vi "find_fiducial_test.vi"() -> ()   [LabVIEW 2019]
uses:
  gVision/gVision.lvlib
  <vilib>/vision/NI_Vision_Development_Module.lvlib
panel:
  out "error out":errorcluster
  out "coords":cluster{"x":dbl, "y":dbl}[](array[cluster])
  out "Image":T1(plugin-control)
  in  "interactive":bool
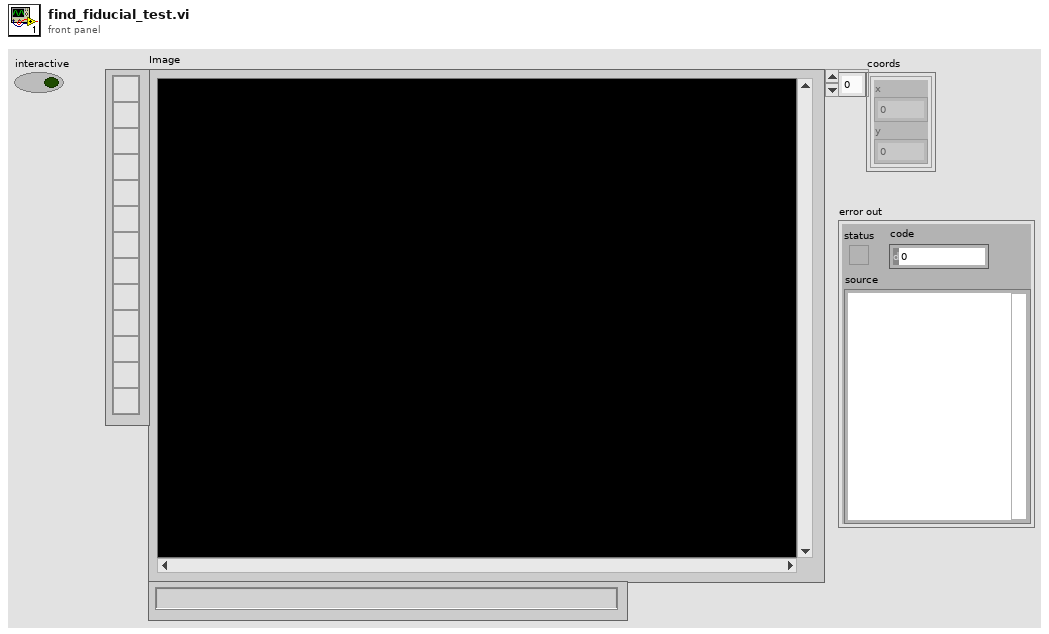
[diagram p1: front panel]
types:
  T1 = typedef "IMAQ Image.ctl" = refnum<image>
  T2 = typedef "Image Type" = u32
  T3 = cluster{"shrinkFactor":sgl, "dilateSize":i32, "sizeMin":sgl, "sizeMax":sgl, "arMin":sgl, "arMax":sgl, "colorGroups":i32, "maxAttempts":i32}
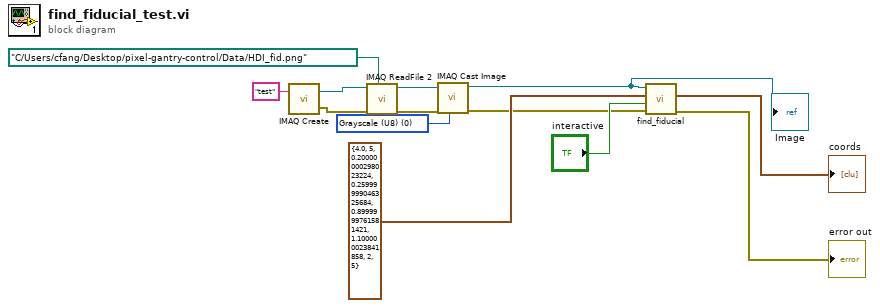
[diagram p0: block diagram]
diagram:
  w1 = T2 0 items=["Grayscale (U8)", "Grayscale (I16)", "Grayscale (SGL)", "Complex (CSG)", "RGB (U32)", "HSL (U32)", "RGB (U64)", "Grayscale (U16)"] ("Image Type")
  n1 = call "IMAQ Create"("Image Name"="test") -> ("New Image"=w11:T1, "error out"=w9:errorcluster)  [unwired: 4 in]
  n2 = call "IMAQ ReadFile 2"("File Path"=path "C:/Users/cfang/Desktop/pixel-gantry-control/Data/HDI_fid.png", "error in (no error)"=w9, "Image"=w11) -> ("error out"=w5:errorcluster, "Image Out"=w3:T1)  [unwired: 4 in, 3 out]
  n3 = call "IMAQ Cast Image"("Image Type"=w1, "error in (no error)"=w5, "Image Src"=w3) -> ("error out"=w4:errorcluster, "Image Dst Out"=w2:T1)  [unwired: 7 in]
  "Image" <- w2
  n4 = call "find_fiducial.vi"("error in"=w4, "interactive"="interactive", "Fiducial Parameters"=T3 {"shrinkFactor"=4.0, "dilateSize"=5, "sizeMin"=0.2, "sizeMax"=0.26, "arMin"=0.9, "arMax"=1.1, "colorGroups"=2, "maxAttempts"=5}, "Image"=w2) -> ("error out"=→"error out":errorcluster, "coords"=→"coords":cluster{"x":dbl, "y":dbl}[])  [unwired: 6 in]
